vi "VICI Release Pump.vi"(8 "error in (no error)":errorcluster, 11 "VISA # in":string) -> (0 "error out":errorcluster, 3 "VISA # out":string)   [LabVIEW 2018, in "VICI M6 M50 Party Mode.lvlib" / "VICI Global Library.lvlib"]
uses:
  VICI Global Library.lvlib
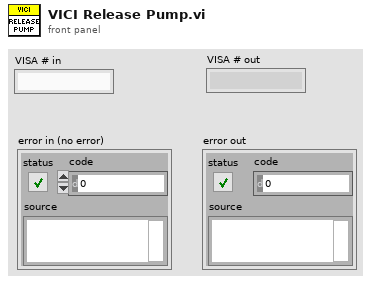
[diagram p1: front panel]
types:
  T1 = cluster{"Busy":bool, "VISA #":string, "Current Pump":string, "Current Function":string, "Pump Array":string[], "Last Success":timestamp, "ID Queue":string[]}[]
  T2 = cluster{"Busy":bool, "VISA #":string, "Current Pump":string, "Current Function":string, "Pump Array":string[], "Last Success":timestamp, "ID Queue":string[]}
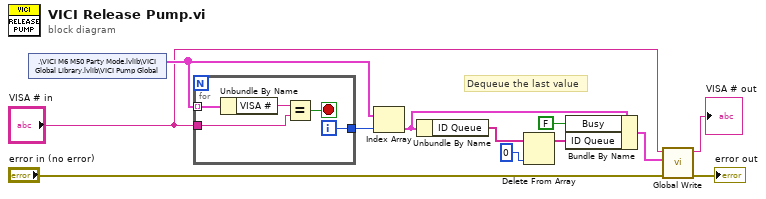
[diagram p0: block diagram]
diagram:
  # "Dequeue the last value"
  n1 = shared-variable ".\\VICI M6 M50 Party Mode.lvlib\\VICI Global Library.lvlib\\VICI Pump Global"() -> (w7:T1)  [unwired: 1 in, 1 out]
  n2 = for {
    tunnel: w7 -> [w17] mode=indexing
    tunnel: "VISA # in" -> [w15]
    tunnel: [w13] -> w5
    i -> [w13]
    stop <- w14 stop-if-true
    n3 = Unbundle By Name(w17) -> ("VISA #"=w16:string)
    n4 = Equal?(x=w16, y=w15) -> (x = y?=w14:bool)
  }
  n5 = Index Array(array=w7, index=w5) -> (element=w3:T2)
  n6 = Unbundle By Name(w3) -> ("ID Queue"=w2:string[])
  n7 = Delete From Array(array=w2, index=0) -> (array with subset deleted=w1:string[])  [unwired: 1 in, 1 out]
  n8 = Bundle By Name(cluster=w3, "Busy"=FALSE, "ID Queue"=w1) -> (w9:T2)
  n9 = call "Global Write.vi"("error in (no error)"="error in (no error)", "VICI Global"=w9, "VISA # in"="VISA # in") -> ("error out"=→"error out":errorcluster, "VISA # out"=→"VISA # out":string)  [unwired: 7 in]
